vi "Configure Trigger.vi"(6 "Delay (0.0 s)":dbl, 8 "error in (no error)":errorcluster, 9 "Slope (0: Positive)":u16(ring) items=["Positive", "Negative"], 10 "Trigger Source (0: Internal)":u16(ring) items=["Internal", "External", "Software (bus)"], 11 "VISA resource name":refnum<visa-resource-name>) -> (0 "error out":errorcluster, 3 "VISA resource name out":refnum<visa-resource-name>)   [LabVIEW 2020, in "AWG.lvlib" / "Agilent 33XXX Series.lvlib"]
doc: "Configures the trigger source for triggering sweeps.\n\n<B>Note</B> This VI does not check the instrument status. If you want to check the instrument status, call the <B>Error Query VI</B> at the conclusion of your sweep operation."
uses:
  Agilent 33XXX Series.lvlib
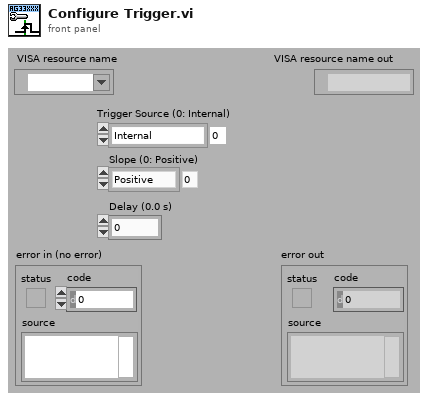
[diagram p1: front panel]
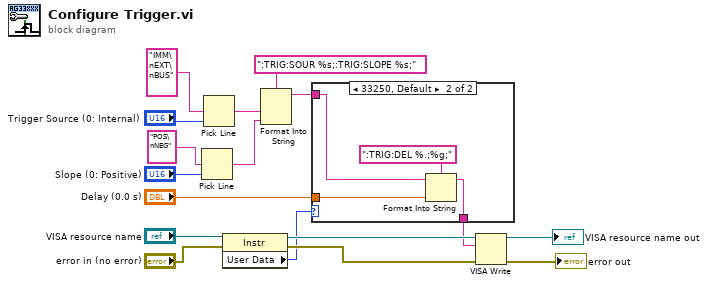
[diagram p0: block diagram]
diagram:
  n1 = Pick Line(multi-line string="POS\nNEG", line index="Slope (0: Positive)") -> (output string=w12:string)  [unwired: 1 in]
  n2 = Pick Line(multi-line string="IMM\nEXT\nBUS", line index="Trigger Source (0: Internal)") -> (output string=w15:string)  [unwired: 1 in]
  n3 = property class="Instr"(reference="VISA resource name", error in="error in (no error)") -> (reference out=w10:refnum<visa-resource-name>, error out=w9:errorcluster, "User Data"=w6:u32)
  n4 = Format Into String(format string=":TRIG:SOUR %s;:TRIG:SLOPE %s;", w15, w12) -> (resulting string=w8:string)  [unwired: 2 in, 1 out]
  n5 = case shown="33250, Default" w6 {
    tunnel: w8 -> [w18 w21]
    tunnel: "Delay (0.0 s)" -> [_ w20]
    tunnel: [w18 w19] -> w5
    frame 33120, 33210, 33220 {
      # "33120,33210 and 33220 models\ndon't support trigger delay"
    }
    frame 33250, Default {
      n6 = Format Into String(format string=":TRIG:DEL %.;%g;", initial string=w21, w20) -> (resulting string=w19:string)  [unwired: 1 in, 1 out]
    }
  }
  n7 = VISA Write(VISA resource name=w10, write buffer=w5, error in (no error)=w9) -> (VISA resource name out=→"VISA resource name out":refnum<visa-resource-name>, error out=→"error out":errorcluster)  [unwired: 1 out]
